vi "SubVREntry.vi"() -> (0 "DataValid":bool, 1 "Value 2":dbl, 2 "VR 2":ext)   [LabVIEW 2020]
panel:
  in  "Cancel Button":bool
  in  "OK Button":bool
  in  "Value":dbl
  in  "VR":ext
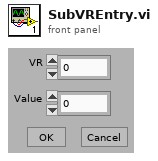
[diagram p1: front panel]
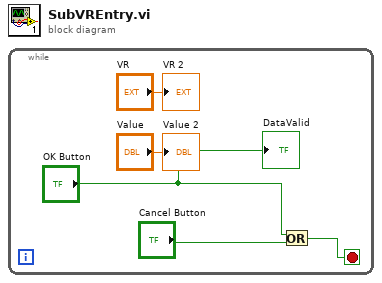
[diagram p0: block diagram]
diagram:
  n1 = while {
    stop <- w5 stop-if-true
    n2 = Or(x="OK Button", y="Cancel Button") -> (x .or. y?=w5:bool)
    "DataValid" <- "OK Button"
    "VR 2" <- "VR"
    "Value 2" <- "Value"
  }
